vi "Map Numeric Representation.vi"(10 "type":T1) -> (2 "representation":T2)   [LabVIEW 2021, in "NI Measurement V2 Client Generator Runtime.lvlib"]
uses:
  NI Measurement V2 Client Generator Runtime.lvlib
  <vilib>/numeric/LVNumericRepresentation.ctl
  <vilib>/gRPC/Generated APIs/ni/measurementlink/measurement/v2/Measurement Service Client V2/RPC Messages/google_protobuf_Field_Kind.ctl
  <vilib>/gRPC/Generated APIs/ni/measurementlink/measurement/v2/Measurement Service Client V2/Measurement Service Client V2.lvlib
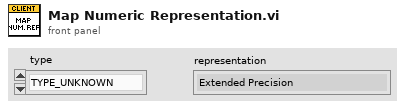
[diagram p1: front panel]
types:
  T1 = typedef "Measurement Service Client V2.lvlib/google_protobuf_Field_Kind.ctl" = enum32{"TYPE_UNKNOWN", "TYPE_DOUBLE", "TYPE_FLOAT", "TYPE_INT64", "TYPE_UINT64", "TYPE_INT32", "TYPE_FIXED64", "TYPE_FIXED32", "TYPE_BOOL", "TYPE_STRING", "TYPE_GROUP", "TYPE_MESSAGE", "TYPE_BYTES", "TYPE_UINT32", "TYPE_ENUM", "TYPE_SFIXED32", "TYPE_SFIXED64", "TYPE_SINT32", "TYPE_SINT64"}
  T2 = typedef "LVNumericRepresentation.ctl" = enum32{"Extended Precision", "Double Precision", "Single Precision", "Long", "Word", "Byte", "Unsigned Long", "Unsigned Word", "Unsigned Byte", "Complex Extended", "Complex Double", "Complex Single", "Quad", "Unsigned Quad", "Fixed-Point"}
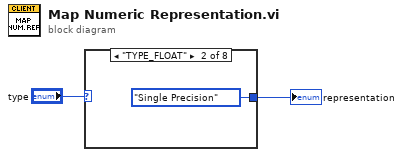
[diagram p0: block diagram]
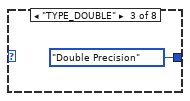
[diagram p3: hidden frame]
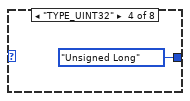
[diagram p4: hidden frame]
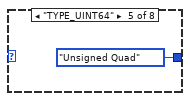
[diagram p5: hidden frame]
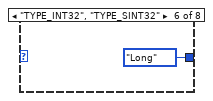
[diagram p6: hidden frame]
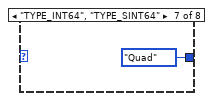
[diagram p7: hidden frame]
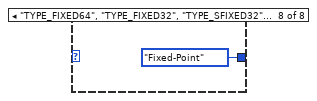
[diagram p8: hidden frame]
diagram:
  n1 = case shown="\"TYPE_FLOAT\"" "type" {
    tunnel: [_ LVNumericRepresentation."Single Precision" ("Representation") LVNumericRepresentation."Double Precision" ("Representation") LVNumericRepresentation."Unsigned Long" ("Representation") LVNumericRepresentation."Unsigned Quad" ("Representation") LVNumericRepresentation."Long" ("Representation") LVNumericRepresentation."Quad" ("Representation") LVNumericRepresentation."Fixed-Point" ("Representation")] -> w2
    frame Default {
    }
    frame "TYPE_FLOAT" {
    }
    frame "TYPE_DOUBLE" {
    }
    frame "TYPE_UINT32" {
    }
    frame "TYPE_UINT64" {
    }
    frame "TYPE_INT32", "TYPE_SINT32" {
    }
    frame "TYPE_INT64", "TYPE_SINT64" {
    }
    frame "TYPE_FIXED64", "TYPE_FIXED32", "TYPE_SFIXED32", "TYPE_SFIXED64" {
    }
  }
  "representation" <- w2
